vi "MacroInterpreterServer_MD.vi"() -> ()   [LabVIEW 2012]
panel:
  in  "stop":bool
  out "remote port":u16
  out "remote address":string
  out "Error Out":errorcluster
  in  "Error In":errorcluster
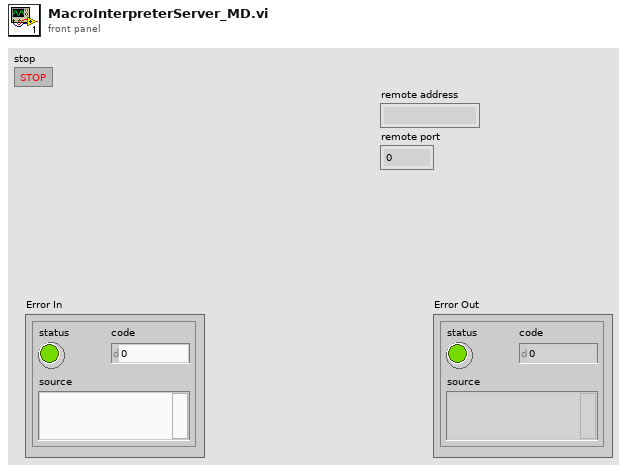
[diagram p1: front panel]
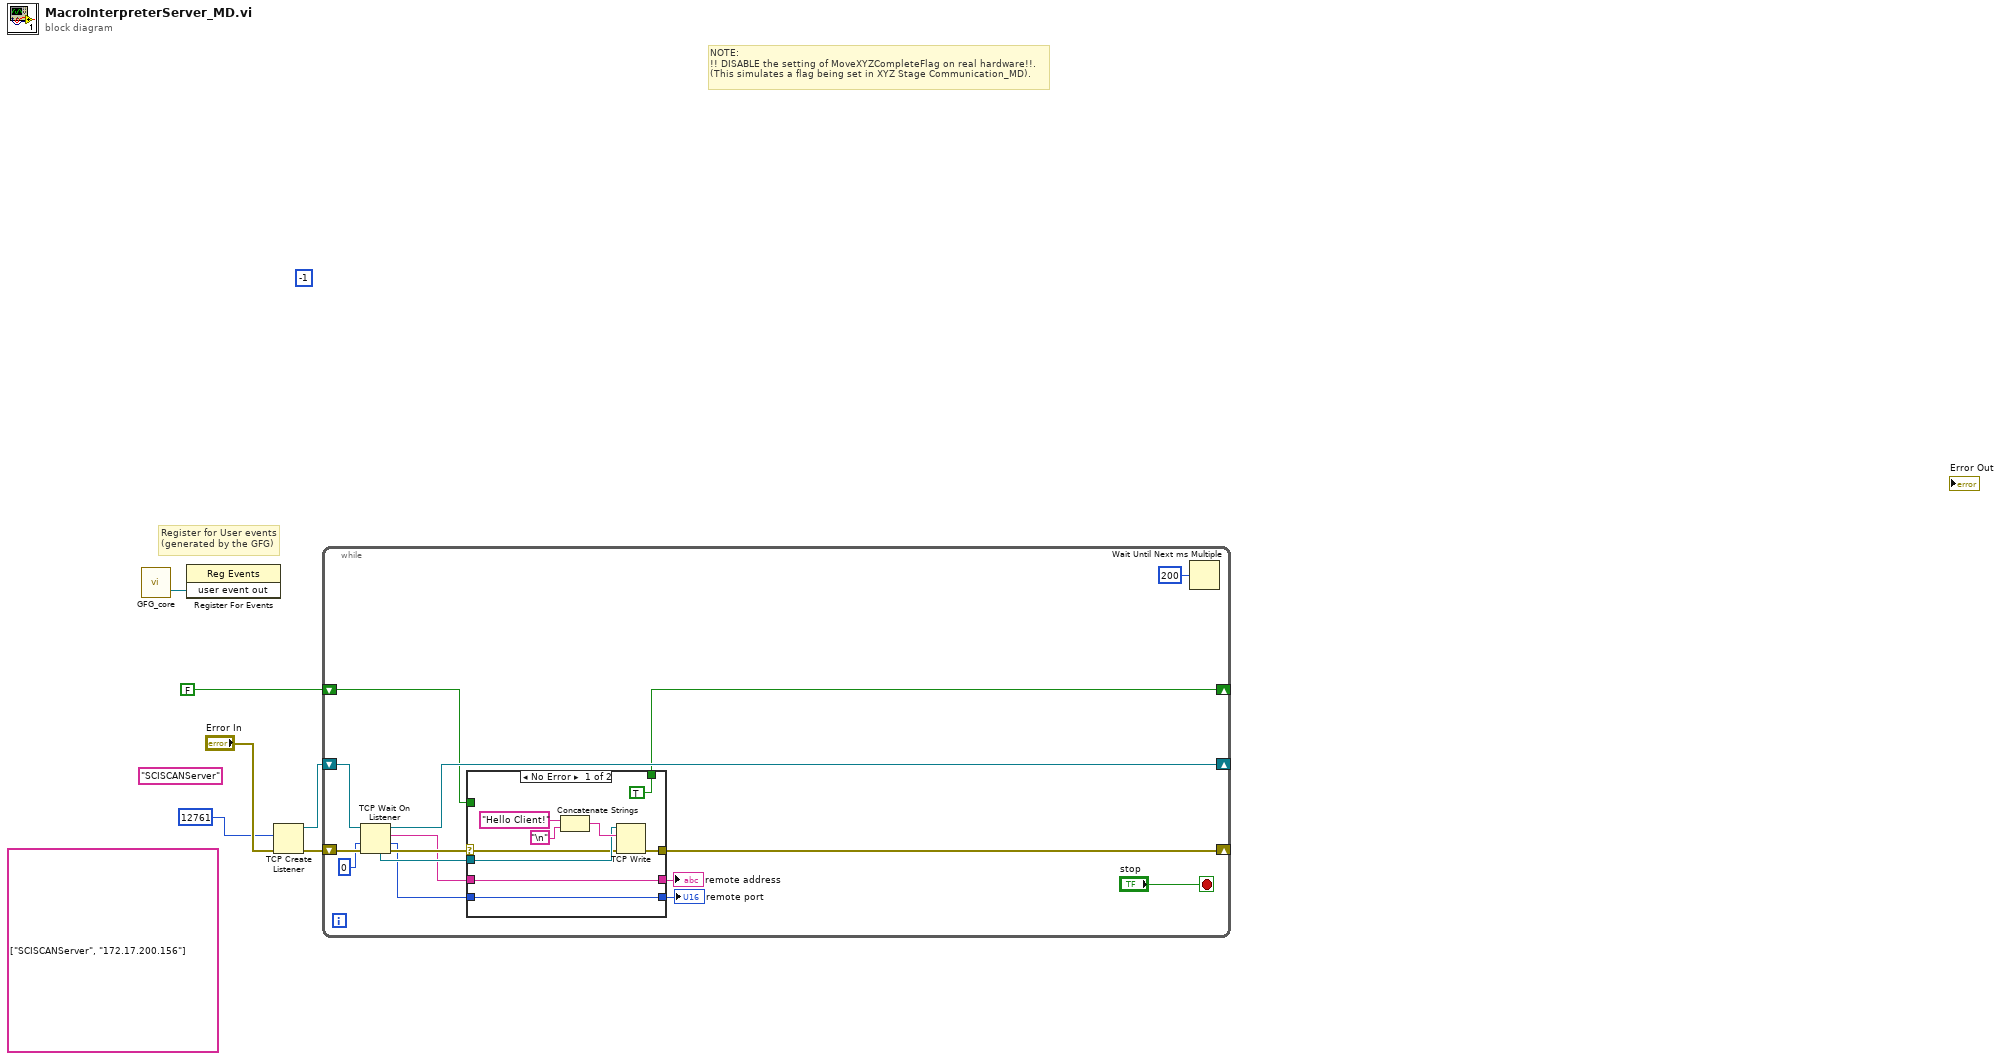
[diagram p0: block diagram]
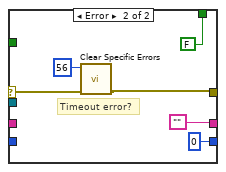
[diagram p2: hidden frame]
diagram:
  (unwired) string[][] [["SCISCANServer", "172.17.200.156"]]
  (unwired) "SCISCANServer" ("service name")
  (unwired) -1
  # "NOTE:\n!! DISABLE the setting of MoveXYZCompleteFlag on real hardware!!.\n(This simulates a flag being set in XYZ Stage Communication_MD)."
  # "Register for User events\n(generated by the GFG)"
  n1 = call "GFG_core.vi"() -> ("user event out"=w6:refnum<user-event>)  [unwired: 13 in, 6 out]
  n2 = register-events(w6) -> ()  [unwired: 2 in, 2 out]
  n3 = TCP Create Listener(8:"Error In", 10:u16 12761 ("port")) -> (0:w4:errorcluster, 3:w3:refnum<k5>)  [unwired: 3 in, 1 out]
  n4 = while {
    shift-right: [w17] -> _
    shift-left: w4 -> [w21]
    shift-right: [w19] -> _
    shift-left: w3 -> [w20]
    shift-right: [w7] -> _
    shift-left: FALSE -> [w8]
    stop <- "stop" stop-if-true
    n5 = TCP Wait On Listener(8:w21, 9:0 ("timeout ms (wait forever: -1)"), 11:w20) -> (0:w13:errorcluster, 1:w11:u16, 2:w12:string, 3:w19:refnum<k5>, 4:w18:refnum<k5>)  [unwired: 1 in]
    n6 = case shown="No Error" w13 {
      selector: w13 -> [w25 w34]
      tunnel: w18 -> [w26 _]
      tunnel: [w30 w36] -> w17
      tunnel: w12 -> [w24 _]
      tunnel: w11 -> [w23 _]
      tunnel: [w24 ""] -> w10
      tunnel: [w23 u16 0 ("remote port")] -> w9
      tunnel: w8 -> [_ _]
      tunnel: [TRUE FALSE] -> w7
      frame No Error {
        n7 = Concatenate Strings("Hello Client!" ("data in"), "\n") -> (w29:string)
        n8 = TCP Write(connection ID=w26, data in=w29, error in (no error)=w25) -> (error out=w30:errorcluster)  [unwired: 1 in, 2 out]
      }
      frame Error {
        # "Timeout error?"
        n9 = call "Clear Specific Errors.vi"("Error In"=w34, "Error number In"=56) -> ("Error Out"=w36:errorcluster)  [unwired: 8 in, 1 out]
      }
    }
    "remote address" <- w10
    "remote port" <- w9
    n10 = Wait Until Next ms Multiple(millisecond multiple=u32 200) -> ()  [unwired: 1 out]
  }
